vi "GetSampleData.vi"(6 "error in":errorcluster caption="错误输入（无错误）", 7 "TimeOut":dbl, 9 "PanelSplitForDisplay.lvclass":refnum<class "PanelSplitForDisplay.lvclass">) -> (0 "error out":errorcluster caption="错误输出", 1 "Display?":bool, 2 "signal out":waveform(dbl), 3 "PanelSplitForDisplay.lvclass 2":refnum<class "PanelSplitForDisplay.lvclass">, 4 "size(s)":i32)   [LabVIEW 2016, in "PanelSplitForDisplay.lvclass"]
uses:
  PanelSplit/PanelSplitForDisplay.lvclass
  HardWare/Ctrls/HardWare _ Data Queue Manage FGV Operation.ctl
  PanelSplit/PanelDataNode/PanelDataNode.lvclass/PanelDataNode.ctl
  MainUI/Config Display Font Size.vi
  PanelSplit/PanelDataNode/PanelDataNode.lvclass
panel:
  out "Time":u32
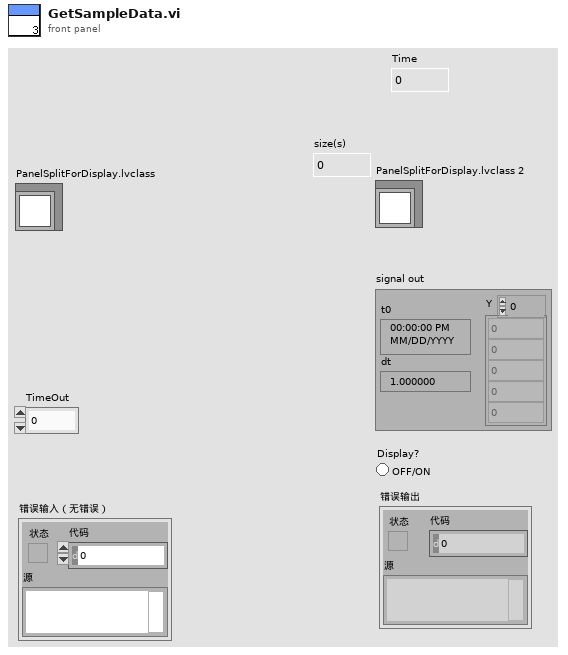
[diagram p1: front panel]
types:
  T1 = typedef "HardWare _ Data Queue Manage FGV Operation.ctl" = enum16{"Initialize", "Add", "Read", "All"}
  T2 = typedef "PanelSplitForDisplay.lvclass/ViValueCtl.ctl" = cluster{"CHTag":string, "GraphProperts":cluster{"YMax":dbl, "YMin":dbl, "ScaleFit":u8}, "CHUnit":string, "CHName":string, "CHValue":string, "CHAlias":string}
  T3 = cluster{"Channel Font Size":u32, "Channel Value Font Size":u32, "Unit Font Size":u32, "Row Font Size":u32, "Display Precision":u32}
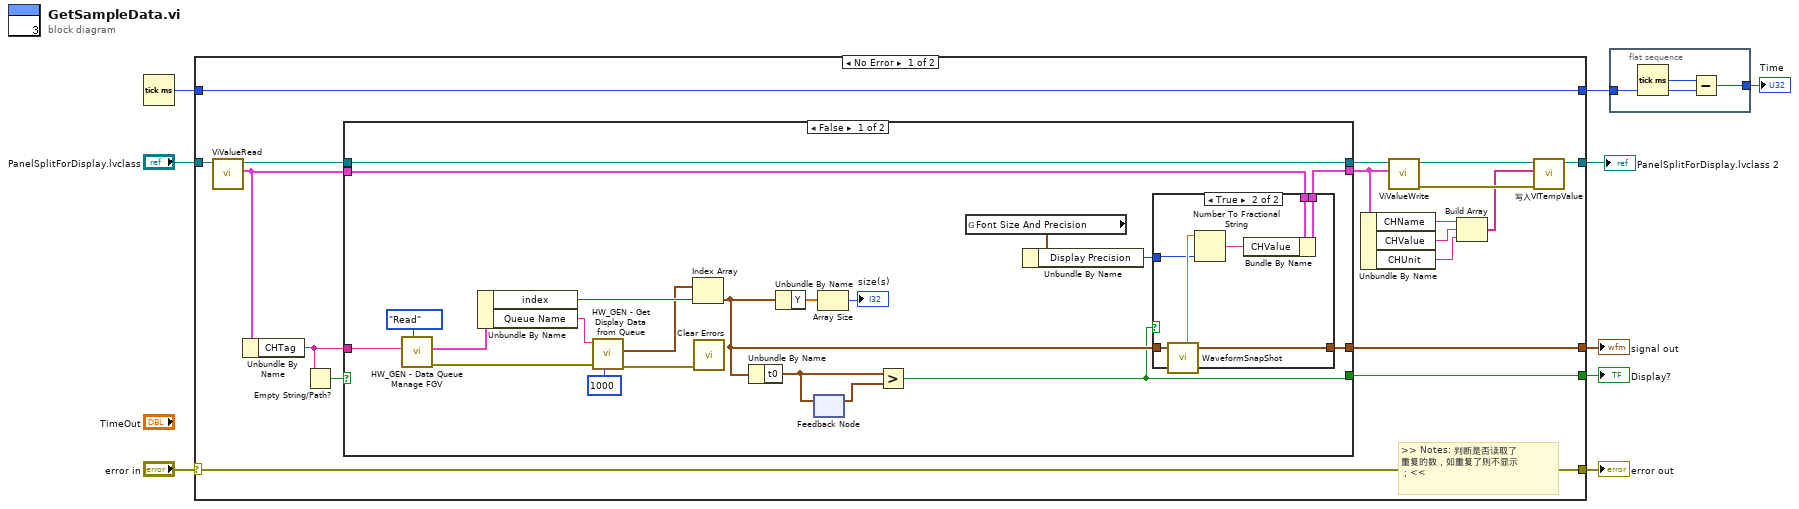
[diagram p0: block diagram]
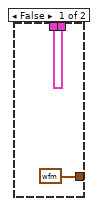
[diagram p2: hidden frame]
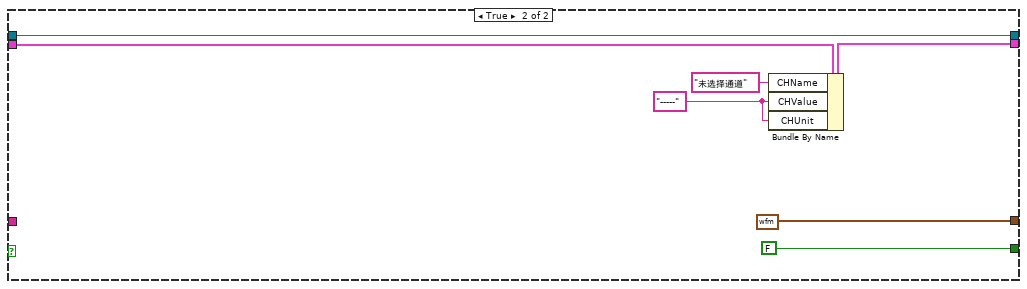
[diagram p3: hidden frame]
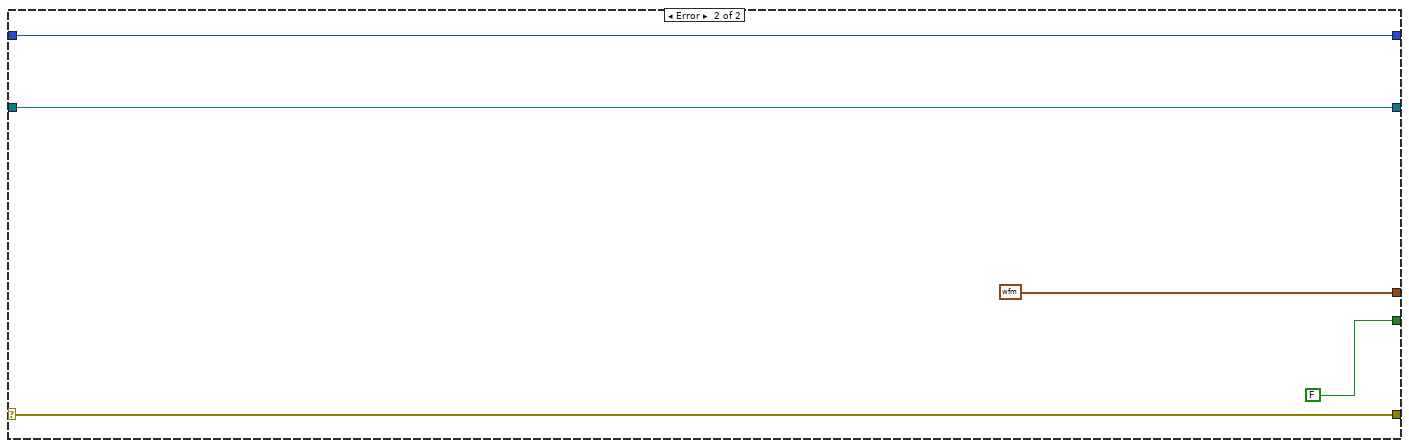
[diagram p4: hidden frame]
diagram:
  n1 = Tick Count (ms)() -> (millisecond timer value=w3:u32)
  n2 = case shown="No Error" "error in" {
    selector: "error in" -> [w27 w69]
    tunnel: [w27 w69] -> w8
    tunnel: "PanelSplitForDisplay.lvclass" -> [w24 w68]
    tunnel: [w18 w68] -> w7
    tunnel: [w25 waveform(dbl) {"t0"=timestamp(0 s since 1904-01-01), "dt"=1.0, "Y"=[]} ("Waveform")] -> w5
    tunnel: [w11 FALSE] -> w4
    tunnel: w3 -> [w10 w65]
    tunnel: [w10 w65] -> w2
    frame No Error {
      # ">> Notes: 判断是否读取了\n重复的数，如重复了则不显示\n；<<"
      n3 = call "ViValueRead.vi"("PanelSplitForDisplay 输入"=w24) -> ("ViValue"=w20:T2, "PanelSplitForDisplay 输出"=w23:refnum<class "PanelSplitForDisplay.lvclass">)  [unwired: 8 in, 1 out]
      n4 = Unbundle By Name(w20) -> ("CHTag"=w22:string)
      n5 = Empty String/Path?(string/path=w22) -> (empty?=w26:bool)
      n6 = case shown="False" w26 {
        tunnel: [w42 waveform(dbl) {"t0"=timestamp(0 s since 1904-01-01), "dt"=1.0, "Y"=[]} ("signal out")] -> w25
        tunnel: w23 -> [w48 w63]
        tunnel: [w48 w63] -> w21
        tunnel: w22 -> [w47 _]
        tunnel: w20 -> [w46 w62]
        tunnel: [w45 w61] -> w16
        tunnel: [w43 FALSE] -> w11
        frame False {
          n7 = call "HW_GEN - Data Queue Manage FGV.vi"("Oper."=HardWare___Data_Queue_Manage_FGV_Operation."Read", "ChanTag"=w47) -> ("error out"=w38:errorcluster, "ChanInfo"=w37:cluster{"Queue Name":string, "index":i32})  [unwired: 7 in, 1 out]
          n8 = Unbundle By Name(w37) -> ("index"=w35:i32, "Queue Name"=w36:string)
          n9 = call "HW_GEN - Get Display Data from Queue.vi"("Time Out(-1)"=1000, "error in"=w38, "Object Name"=w36) -> ("error out"=w34:errorcluster, "data"=w31:waveform(dbl)[])  [unwired: 6 in, 1 out]
          n10 = Index Array(array=w31, index=w35) -> (element=w44:waveform(dbl))
          n11 = call <vilib>:"Clear Errors.vi"("error in (no error)"=w34) -> ()  [unwired: 5 in, 2 out]
          n12 = Unbundle By Name(w44) -> ("t0"=w30:timestamp)
          n13 = Unbundle By Name(w44) -> ("Y"=w29:dbl[])
          n14 = feedback #1() -> (w33:timestamp)  [unwired: 1 in]
          n15 = feedback-in #1(w30) -> ()
          n16 = Array Size(array=w29) -> (size(s)=→"size(s)":i32)
          n17 = Greater?(x=w30, y=w33) -> (0:w43:bool)
          n18 = global read "Config Display Font Size.vi" "Font Size And Precision"() -> (w41:T3)
          n19 = Unbundle By Name(w41) -> ("Display Precision"=w40:u32)
          n20 = case shown="True" w43 {
            tunnel: w46 -> [w50 w57]
            tunnel: [w50 w55] -> w45
            tunnel: w44 -> [_ w54]
            tunnel: [waveform(dbl) {"t0"=timestamp(0 s since 1904-01-01), "dt"=1.0, "Y"=[]} ("signal out") w53] -> w42
            tunnel: w40 -> [_ w51]
            frame False {
            }
            frame True {
              n21 = call "WaveformSnapShot.vi"("RawWave"=w54) -> ("Mean"=w52:dbl, "SnapWave"=w53:waveform(dbl))  [unwired: 7 in]
              n22 = Number To Fractional String(number=w52, precision (6)=w51) -> (F-format string=w56:string)  [unwired: 2 in]
              n23 = Bundle By Name(cluster=w57, "CHValue"=w56) -> (w55:T2)
            }
          }
        }
        frame True {
          w59 = "-----" ("Channel")
          n24 = Bundle By Name(cluster=w62, "CHName"="未选择通道", "CHValue"=w59, "CHUnit"=w59) -> (w61:T2)
        }
      }
      n25 = Unbundle By Name(w16) -> ("CHName"=w15:string, "CHValue"=w14:string, "CHUnit"=w13:string)
      n26 = call "ViValueWrite.vi"("ViValue"=w16, "PanelSplitForDisplay 输入"=w21) -> ("error out"=w17:errorcluster, "PanelSplitForDisplay 输出"=w19:refnum<class "PanelSplitForDisplay.lvclass">)  [unwired: 8 in]
      n27 = Build Array(w15, w14, w13) -> (w12:string[])
      n28 = call "写入VITempValue.vi"("error in (no error)"=w17, "VITempValue"=w12, "PanelDataNode输入"=w19) -> ("PanelDataNode输出"=w18:refnum<class "PanelSplitForDisplay.lvclass">)  [unwired: 7 in, 1 out]
    }
    frame Error {
    }
  }
  "error out" <- w8
  "signal out" <- w5
  "PanelSplitForDisplay.lvclass 2" <- w7
  "Display?" <- w4
  n29 = flat-sequence {
    tunnel: w2 -> [w72]
    tunnel: [w70] -> w1
    frame #0 {
      n30 = Tick Count (ms)() -> (millisecond timer value=w71:u32)
      n31 = Subtract(x=w71, y=w72) -> (x-y=w70:u32)
    }
  }
  "Time" <- w1
